vi "FPGA Threshold (Under).vi"(7 "number of channels":T2=1 items=["1"=1, "2"=2, "3"=3, "4"=4, "5"=5, "6"=6, "7"=7, "8"=8, "9"=9, "10"=10, "11"=11, "12"=12, "13"=13, "14"=14, "15"=15, "16"=16], 9 "input valid? (T)":bool=TRUE, 10 "pick-up settings":T1, 11 "G":fxp<+/-,48,24>) -> (0 "error":i32, 1 "output valid?":bool, 3 "pick-up signal?":bool)   [LabVIEW 2013, in "NI_EP_Protection_FPGA.lvlib"]
doc: "Detects the input energizing quantity <B>G</B> for deciding whether <B>G</B> turns to a pick-up signal according to <B>pick-up settings</B>."
uses:
  <vilib>/addons/Electrical Power/Protection/NI_EP_Protection_FPGA.lvlib
  <vilib>/addons/Electrical Power/PQ/Resampling/FPGA/subVIs/fpga_NofCH.ctl
  <vilib>/addons/Electrical Power/Protection/Threshold/subVIs/fpga_Pick-up Setting.ctl
  <vilib>/addons/Electrical Power/PQ/Resampling/NI_EP_Resample_FPGA.lvlib
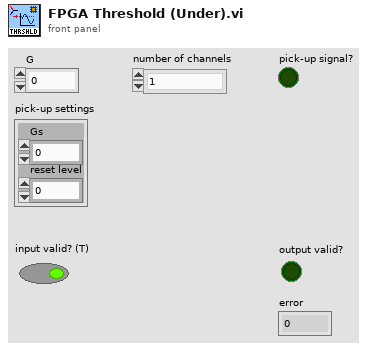
[diagram p1: front panel]
types:
  T1 = typedef "NI_EP_Protection_FPGA.lvlib/fpga_pick-up setting.ctl" = cluster{"Gs":fxp<+/-,48,24>, "reset level":fxp<+/-,48,24>}
  T2 = typedef "NI_EP_Resample_FPGA.lvlib/fpga_NofCH.ctl" = u8
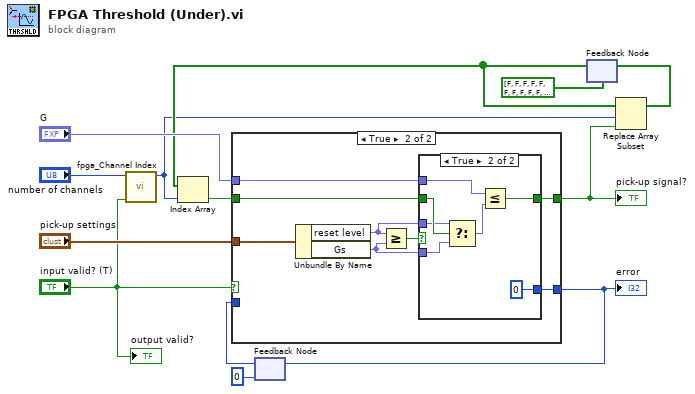
[diagram p0: block diagram]
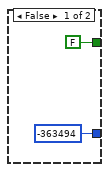
[diagram p3: hidden frame]
diagram:
  n1 = call <vilib>:"fpga_Channel Index.vi"("input valid? (T)"="input valid? (T)", "number of channels"="number of channels") -> ("channel index"=w6:u8)  [unwired: 9 in]
  n2 = feedback #1(0 ("code")) -> (w2:i32)
  n3 = feedback #2(bool[] [FALSE, FALSE, FALSE, FALSE, FALSE, FALSE, FALSE, FALSE, FALSE, FALSE, FALSE, FALSE, FALSE, FALSE, FALSE, FALSE]) -> (w8:bool[])
  n4 = Index Array(array=w8, index=w6) -> (element=w7:bool)
  n5 = case shown="True" "input valid? (T)" {
    tunnel: [w15 w21] -> w1
    tunnel: "G" -> [_ w22]
    tunnel: "pick-up settings" -> [_ w20]
    tunnel: w7 -> [w15 w23]
    tunnel: [w14 w18] -> w3
    tunnel: w2 -> [w14 _]
    frame False {
    }
    frame True {
      n6 = Unbundle By Name(w20) -> ("reset level"=w17:fxp<+/-,48,24>, "Gs"=w16:fxp<+/-,48,24>)
      n7 = Greater Or Equal?(x=w17, y=w16) -> (x >= y?=w19:bool)
      n8 = case shown="True" w19 {
        tunnel: w23 -> [_ w32]
        tunnel: w22 -> [_ w31]
        tunnel: [FALSE w29] -> w21
        tunnel: [-363494 ("error") 0 ("error")] -> w18
        tunnel: w17 -> [_ w27]
        tunnel: w16 -> [_ w26]
        frame False {
        }
        frame True {
          n9 = Select(t=w27, s=w32, f=w26) -> (s? t:f=w30:fxp<+/-,48,24>)
          n10 = Less Or Equal?(x=w31, y=w30) -> (x <= y?=w29:bool)
        }
      }
    }
  }
  "pick-up signal?" <- w1
  "error" <- w3
  n11 = feedback-in #1(w3) -> ()
  n12 = Replace Array Subset(array=w8, new element=w1, index=w6) -> (w9:bool[])
  n13 = feedback-in #2(w9) -> ()
  "output valid?" <- "input valid? (T)"
